vi "TimeInterpVariant_AddSample.vi"(9 "Variant":variant, 10 "TimeStamp":dbl, 11 "in TimeInterpVariant":T1) -> (0 "Error":bool, 3 "out TimeInterpVariant":T1)   [LabVIEW 2019, in "Trajectory_Library.lvlib"]
doc: "Add a sample to the buffer.\n \nInputs:\n - In TimeInterpPose2d -- Time Interp data cluster \n - Time -- The time stamp of the sample (seconds)\n - Value -- The Pose2d value\n\nOutputs:\n - out TimeInterpPose2d -- Updated Time Interp data cluster"
uses:
  Trajectory_Library.lvlib
  <vilib>/gmath/NI_Gmath.lvlib
  TypeDef/TIME_INTERPOLATABLE_VARIANT.ctl
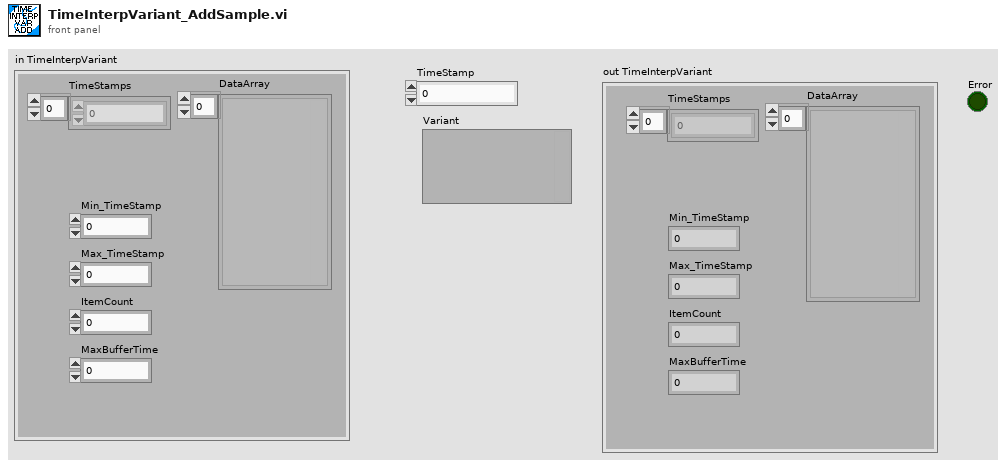
[diagram p1: front panel]
types:
  T1 = typedef "Trajectory_Library.lvlib/TIME_INTERPOLATABLE_VARIANT.ctl" = cluster{"TimeStamps":dbl[], "DataArray":variant[], "Min_TimeStamp":dbl, "Max_TimeStamp":dbl, "ItemCount":i32, "MaxBufferTime":dbl}
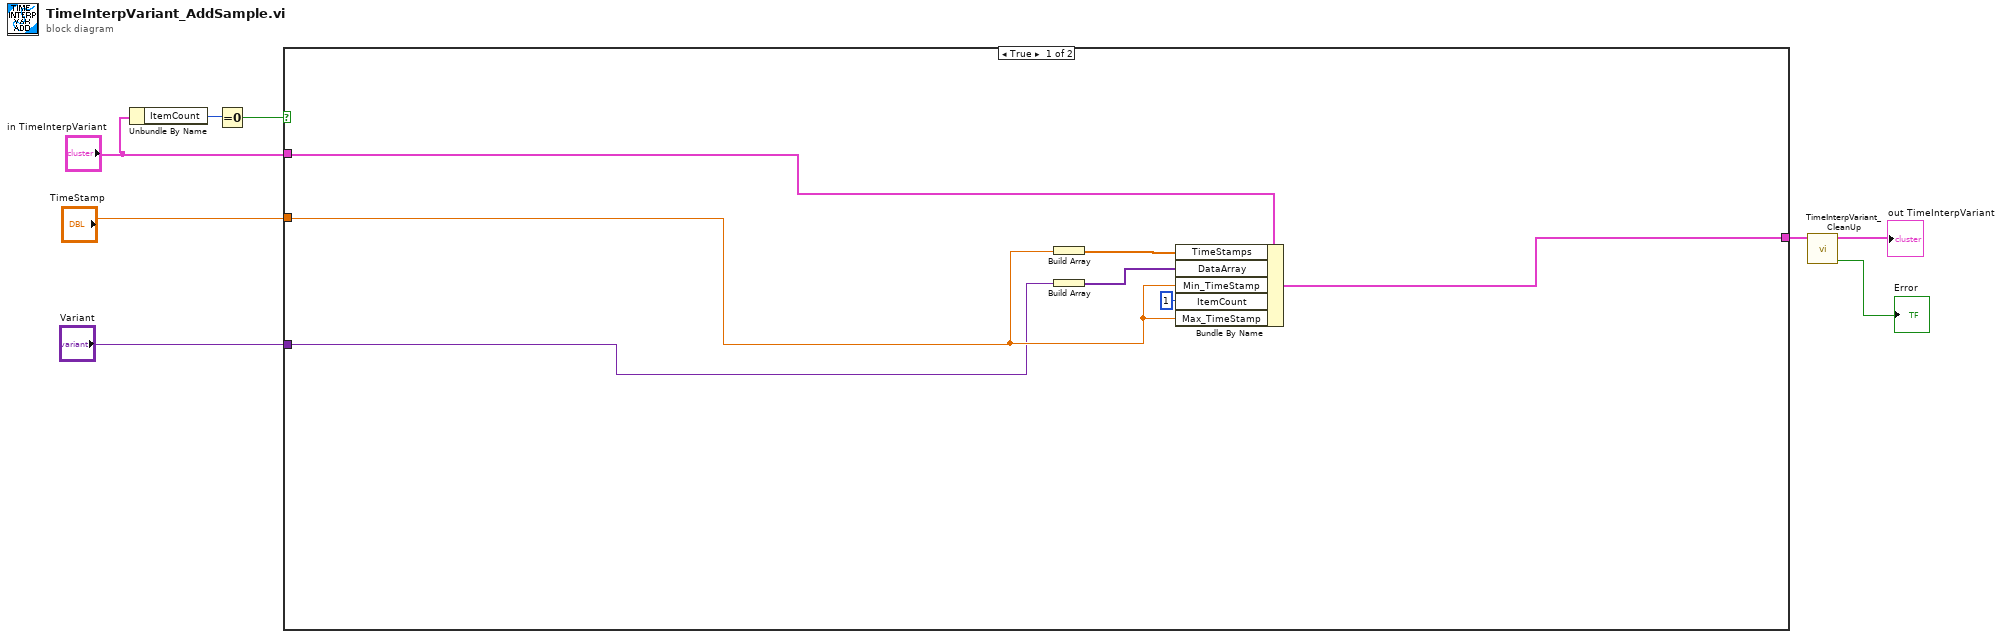
[diagram p0: block diagram]
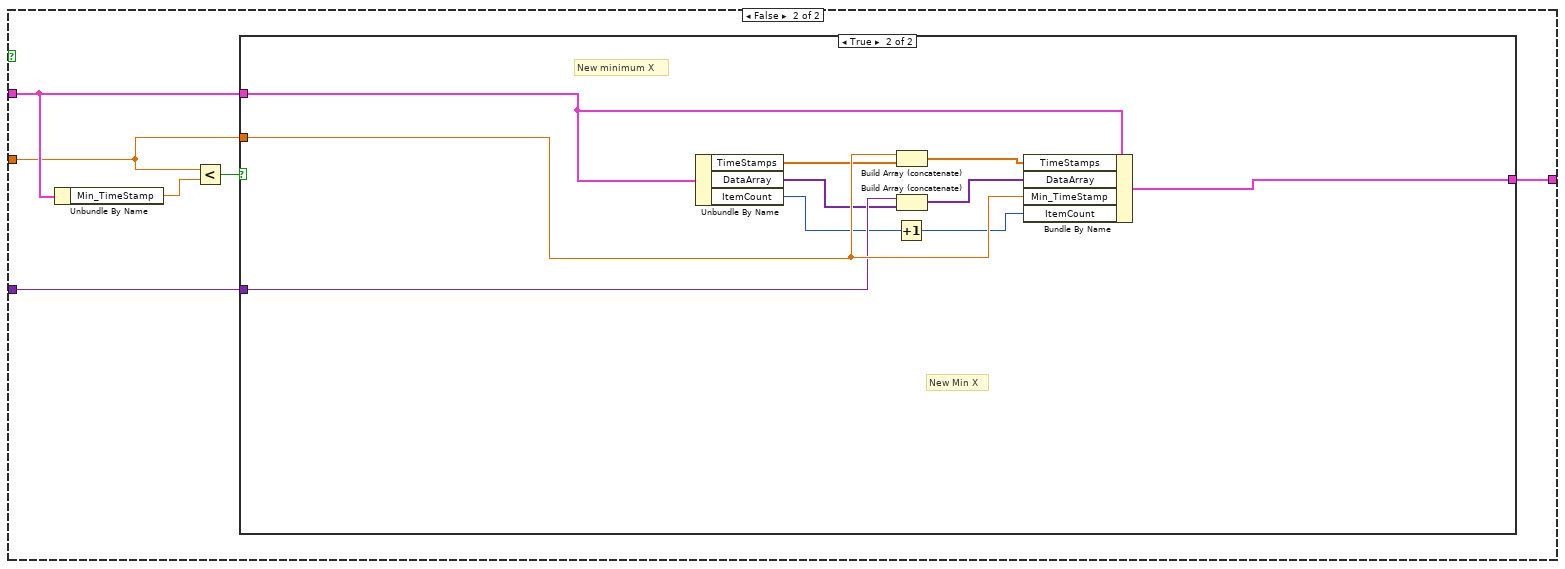
[diagram p2: hidden frame]
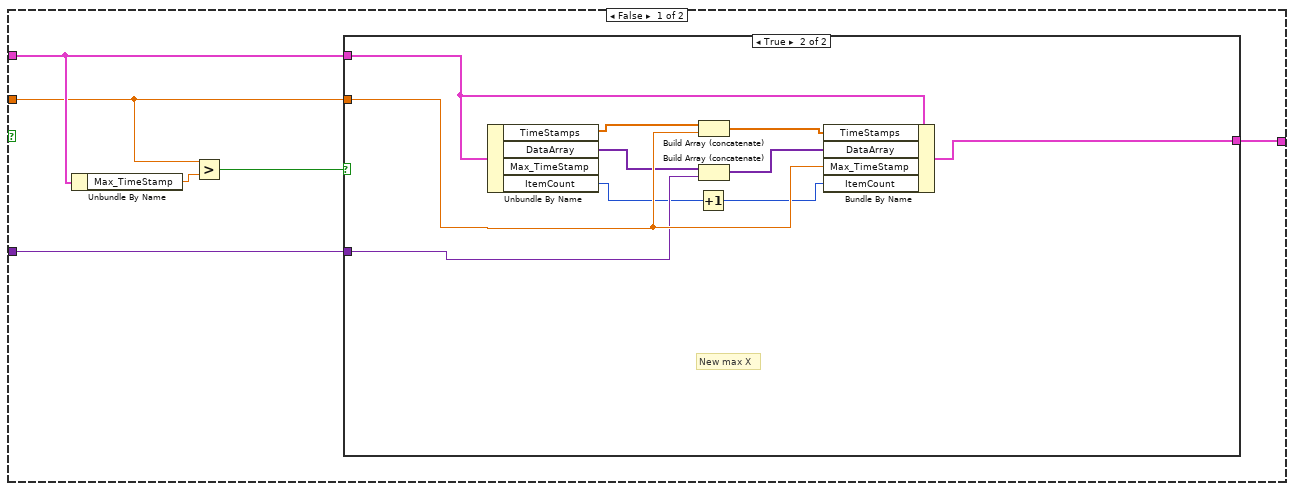
[diagram p3: hidden frame]
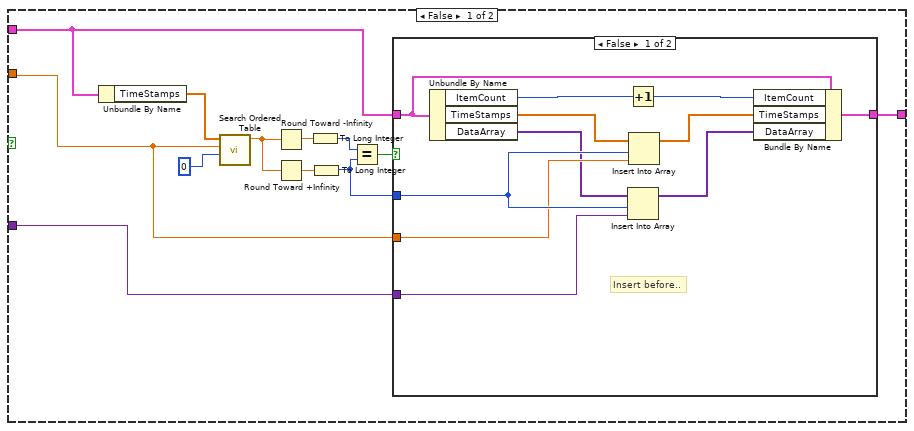
[diagram p4: hidden frame]
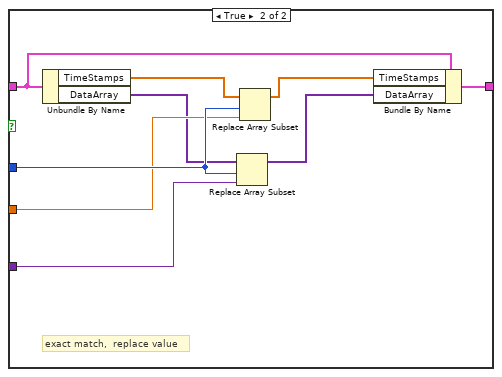
[diagram p5: hidden frame]
diagram:
  n1 = Unbundle By Name("in TimeInterpVariant") -> ("ItemCount"=w3:i32)
  n2 = Equal To 0?(x=w3) -> (x = 0?=w2:bool)
  n3 = case shown="True" w2 {
    tunnel: "in TimeInterpVariant" -> [w15 w19]
    tunnel: "TimeStamp" -> [w14 w18]
    tunnel: "Variant" -> [w13 w17]
    tunnel: [w12 w16] -> w1
    frame True {
      n4 = Build Array(w14) -> (w11:dbl[])
      n5 = Build Array(w13) -> (w10:variant[])
      n6 = Bundle By Name(cluster=w15, "TimeStamps"=w11, "DataArray"=w10, "Min_TimeStamp"=w14, "ItemCount"=1, "Max_TimeStamp"=w14) -> (w12:T1)
    }
    frame False {
      n7 = Unbundle By Name(w19) -> ("Min_TimeStamp"=w21:dbl)
      n8 = Less?(x=w18, y=w21) -> (x < y?=w20:bool)
      n9 = case shown="True" w20 {
        tunnel: w19 -> [w26 w79]
        tunnel: w18 -> [w24 w78]
        tunnel: w17 -> [w23 w77]
        tunnel: [w25 w76] -> w16
        frame False {
          n10 = Unbundle By Name(w26) -> ("Max_TimeStamp"=w27:dbl)
          n11 = Greater?(x=w24, y=w27) -> (0:w22:bool)
          n12 = case shown="True" w22 {
            tunnel: w26 -> [w32 w69]
            tunnel: [w28 w68] -> w25
            tunnel: w24 -> [w30 w67]
            tunnel: w23 -> [w29 w66]
            frame False {
              n13 = Unbundle By Name(w32) -> ("TimeStamps"=w38:dbl[])
              n14 = call <vilib>:"Search Ordered Table.vi"("starting index"=0, "x value"=w30, "ordered x array"=w38) -> ("fractional index"=w37:dbl)  [unwired: 8 in]
              n15 = Round Toward -Infinity(1:w37) -> (0:w35:dbl)
              n16 = Round Toward +Infinity(x=w37) -> (ceil(x): smallest int >= x=w36:dbl)
              n17 = To Long Integer(number=w35) -> (32bit integer=w34:i32)
              n18 = To Long Integer(number=w36) -> (32bit integer=w31:i32)
              n19 = Equal?(x=w34, y=w31) -> (x = y?=w33:bool)
              n20 = case shown="False" w33 {
                tunnel: w32 -> [w47 w59]
                tunnel: w31 -> [w50 w58]
                tunnel: w30 -> [w49 w57]
                tunnel: w29 -> [w48 w56]
                tunnel: [w46 w55] -> w28
                frame False {
                  # "Insert before.."
                  n21 = Unbundle By Name(w47) -> ("ItemCount"=w45:i32, "TimeStamps"=w43:dbl[], "DataArray"=w42:variant[])
                  n22 = Increment(x=w45) -> (x+1=w44:i32)
                  n23 = Insert Into Array(array=w42, index=w50, new element=w48) -> (w40:variant[])
                  n24 = Insert Into Array(array=w43, index=w50, new element=w49) -> (w41:dbl[])
                  n25 = Bundle By Name(cluster=w47, "ItemCount"=w44, "TimeStamps"=w41, "DataArray"=w40) -> (w46:T1)
                }
                frame True {
                  # "exact match,  replace value"
                  n26 = Unbundle By Name(w59) -> ("TimeStamps"=w54:dbl[], "DataArray"=w53:variant[])
                  n27 = Replace Array Subset(array=w53, new element=w56, index=w58) -> (w51:variant[])
                  n28 = Replace Array Subset(array=w54, new element=w57, index=w58) -> (w52:dbl[])
                  n29 = Bundle By Name(cluster=w59, "TimeStamps"=w52, "DataArray"=w51) -> (w55:T1)
                }
              }
            }
            frame True {
              # "New max X"
              n30 = Unbundle By Name(w69) -> ("TimeStamps"=w61:dbl[], "DataArray"=w60:variant[], "ItemCount"=w63:i32)  [unwired: 1 out]
              n31 = Increment(x=w63) -> (x+1=w62:i32)
              n32 = Build Array (concatenate)(w61, w67) -> (w65:dbl[])
              n33 = Build Array (concatenate)(w60, w66) -> (w64:variant[])
              n34 = Bundle By Name(cluster=w69, "TimeStamps"=w65, "DataArray"=w64, "Max_TimeStamp"=w67, "ItemCount"=w62) -> (w68:T1)
            }
          }
        }
        frame True {
          # "New Min X"
          # "New minimum X"
          n35 = Unbundle By Name(w79) -> ("TimeStamps"=w75:dbl[], "DataArray"=w72:variant[], "ItemCount"=w71:i32)
          n36 = Increment(x=w71) -> (x+1=w70:i32)
          n37 = Build Array (concatenate)(w78, w75) -> (w74:dbl[])
          n38 = Build Array (concatenate)(w77, w72) -> (w73:variant[])
          n39 = Bundle By Name(cluster=w79, "TimeStamps"=w74, "DataArray"=w73, "Min_TimeStamp"=w78, "ItemCount"=w70) -> (w76:T1)
        }
      }
    }
  }
  n40 = call "TimeInterpVariant_CleanUp.vi"("in TimeInterpVariant"=w1) -> ("Error"=→"Error":bool, "out TimeInterpVariant"=→"out TimeInterpVariant":T1)  [unwired: 9 in]
